vi "Test_TTL_read.vi"() -> ()   [LabVIEW 2016]
panel:
  out "Notifier error out":errorcluster
  out "VISA error out":errorcluster
  in  "Stop Button":bool
  in  "VISA resource name":refnum<visa-resource-name>="ASRL3::INSTR"
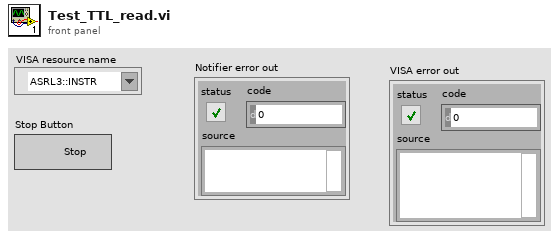
[diagram p1: front panel]
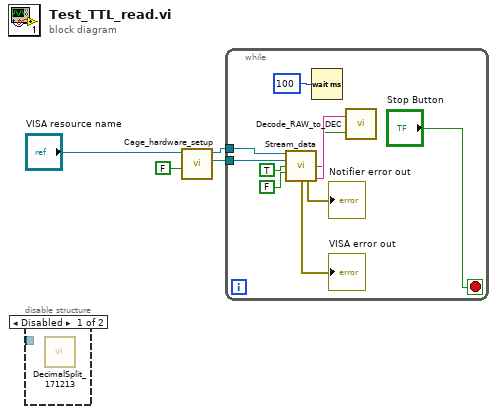
[diagram p0: block diagram]
diagram:
  n1 = disable-structure shown="Disabled" {
    disable-tunnel: _ -> [w5 _]
    frame Disabled {
      n2 = call "DecimalSplit_171213.vi"() -> ()  [unwired: 4 in, 4 out]
    }
    frame Enabled {
    }
  }
  n3 = call "Cage_hardware_setup.vi"("VISA resource name"="VISA resource name", "Close port? (T)"=FALSE) -> ("VISA resource name out"=w3:refnum<visa-resource-name>, "ReadStatus"=w2:refnum<notifier>)  [unwired: 4 in, 3 out]
  n4 = while {
    tunnel: w3 -> [w12]
    tunnel: w2 -> [w11]
    stop <- "Stop Button" stop-if-true
    n5 = call "Stream_data.vi"("VISA resource name in"=w12, "ReadStatus in"=w11, "Play / Pause"=TRUE, "Read TTL status in"=FALSE ("Read TTL status")) -> ("Read TTL status out"=w6:bool, "VISA error out"=→"VISA error out":errorcluster, "Notifier error out"=→"Notifier error out":errorcluster, "read buffer"=w13:string)  [unwired: 5 in, 3 out]
    n6 = Wait (ms)(milliseconds to wait=u32 100) -> ()  [unwired: 1 out]
    n7 = call "Decode_RAW_to_DEC.vi"("Read TTL status"=w6, "read buffer"=w13) -> ()  [unwired: 1 out]
  }
